vi "Library.Close.vi"(8 "error in (no error)":errorcluster, 11 "Library Reference":refnum<vi>) -> (0 "error out":errorcluster)   [LabVIEW 2011]
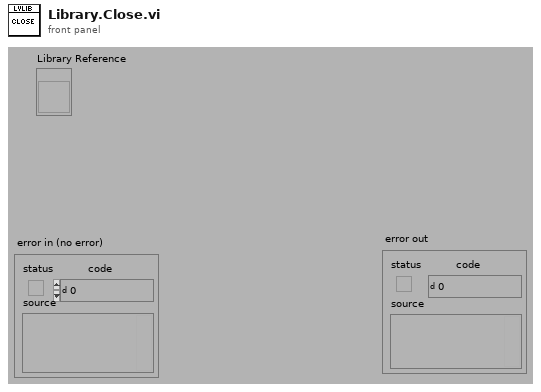
[diagram p1: front panel]
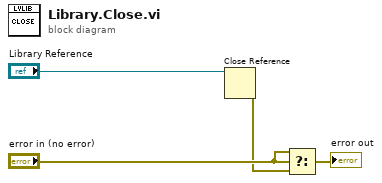
[diagram p0: block diagram]
diagram:
  n1 = Close Reference(reference="Library Reference") -> (error out=w2:errorcluster)  [unwired: 1 in]
  n2 = Select(t="error in (no error)", s="error in (no error)", f=w2) -> (s? t:f=→"error out":errorcluster)
